vi "Agilent 34970 Read Scan List.vi"(8 "error in (no error)":errorcluster, 11 "VISA Resource Name":refnum<visa-resource-name>) -> (0 "error out":errorcluster, 2 "Scan List":string, 3 "VISA Resource Name Out":refnum<visa-resource-name>)   [LabVIEW 2018]
uses:
  Agilent 34970.lvlib
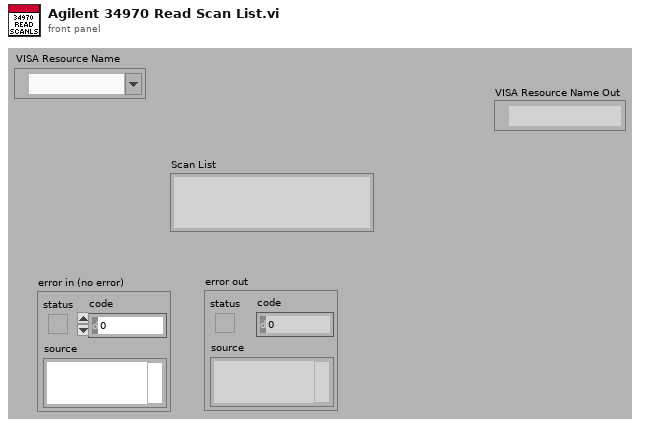
[diagram p1: front panel]
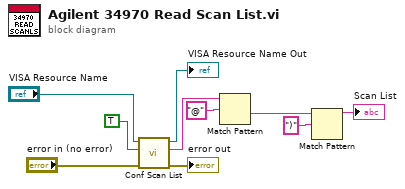
[diagram p0: block diagram]
diagram:
  n1 = call "Conf Scan List.vi"("error in (no error)"="error in (no error)", "Set/Check (F:Set)"=TRUE, "VISA Resource Name"="VISA Resource Name") -> ("error out"=→"error out":errorcluster, "Configuration?"=w5:string, "VISA Resource Name Out"=→"VISA Resource Name Out":refnum<visa-resource-name>)  [unwired: 6 in]
  n2 = Match Pattern(string=w5, regular expression="@") -> (after substring=w3:string)  [unwired: 1 in, 3 out]
  n3 = Match Pattern(string=w3, regular expression=")") -> (before substring=→"Scan List":string)  [unwired: 1 in, 3 out]
